vi "RS485通信实验.vi"   [LabVIEW 2011]
uses:
  <vilib>/STM32_DriverVI_Interface_F4/UART/UART Resource Name_F4.ctl
  <vilib>/STM32_DriverVI_Interface_F4/GPIO/PortX_in_F4.ctl
  <vilib>/STM32_DriverVI_Interface_F4/GPIO/pin_in_F4.ctl
  <vilib>/STM32_DriverVI_Interface_F4/GPIO/GPO_Mode_Interface_F4.ctl
  <vilib>/STM32_DriverVI_Interface_F4/LCD/Show_Mode_F4.ctl
  <vilib>/STM32_DriverVI_Interface_F4/LCD/Font_Size_F4.ctl
  <vilib>/STM32_DriverVI_Interface_F4/LCD/Brush Color_Index_F4.ctl
  <vilib>/eio/EIO_TerminalDirection.ctl
  <vilib>/STM32_DriverVI_Interface_F4/LCD/LCD_Init_F4.vi
  <vilib>/STM32_DriverVI_Interface_F4/GPIO_EIO/GPI_EIO_Inner_F4.vi
  <vilib>/eio/EIONode/EIONode.xnode
types:
  T1 = typedef "GPO_Mode_Interface_F4.ctl" = enum8{"Push-pull Output", "Open-drain Output"}
  T2 = typedef "pin_in_F4.ctl" = enum8{"P0", "P1", "P2", "P3", "P4", "P5", "P6", "P7", "P8", "P9", "P10", "P11", "P12", "P13", "P14", "P15"}
  T3 = typedef "PortX_in_F4.ctl" = enum8{"Port_A", "Port_B", "Port_C", "Port_D", "Port_E", "Port_F", "Port_G", "Port_H", "Port_I"}
  T4 = enum16{"1.0 bit", "0.5 bit", "2.0 bit", "1.5 bit"}
  T5 = enum16{"None parity", "Odd parity", "Even parity"}
  T6 = typedef "UART Resource Name_F4.ctl" = enum8{"COM 1", "COM 2", "COM 3", "COM 4", "COM 5", "COM 6"}
  T7 = typedef "STM32时钟倍频_F4.ctl" = u8
  T8 = typedef "Show_Mode_F4.ctl" = enum8{"非叠加显示", "叠加显示"}
  T9 = typedef "Font_Size_F4.ctl" = enum8{"Small_Font（12）", "Big_Font（16）"}
  T10 = typedef "Brush Color_Index_F4.ctl" = enum8{"White", "Black", "Blue", "Green_Blue", "Red", "Magenta（品红）", "Green", "Cyan（青色）", "Yellow", "Brown", "Brown_Red", "Gray", "Dark_Blue", "Light_Blue", "Gray_Blue", "Light_Green", "Light_Gray", "Light_Gray_Blue", "Light_Brown_Blue"}
  T11 = enum8{"P0", "P1", "P2", "P3", "P4", "P5", "P6", "P7", "P8", "P9", "P10", "P11", "P12", "P13", "P14", "P15"}
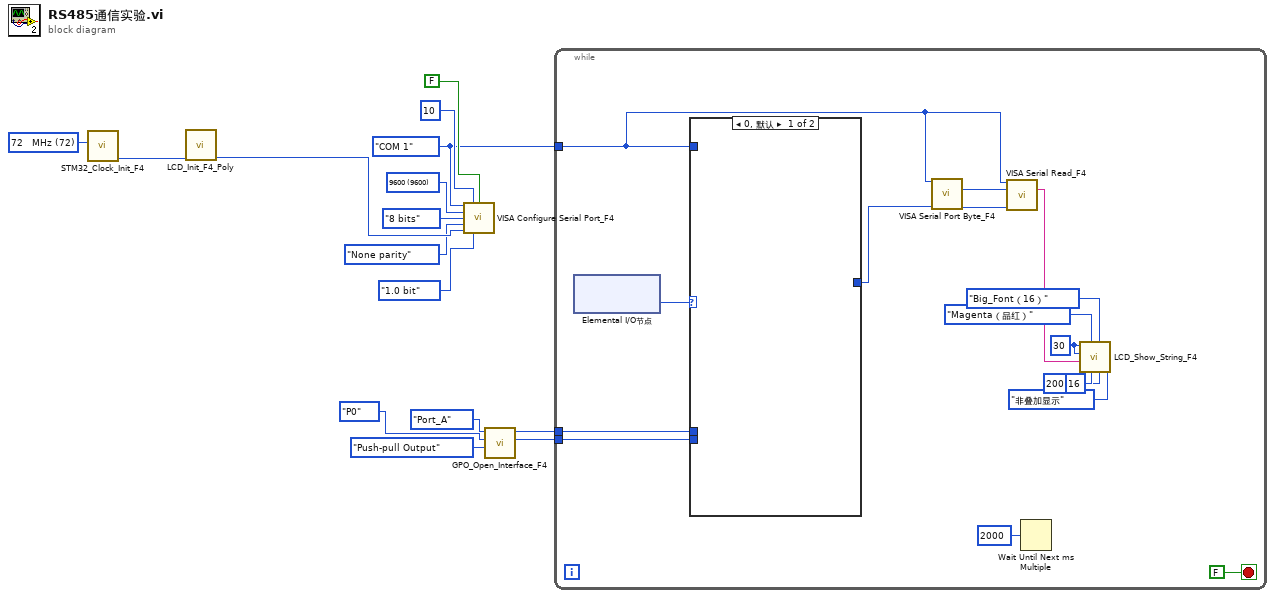
[diagram p0: block diagram]
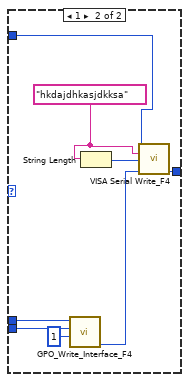
[diagram p2: hidden frame]
diagram:
  w12 = u32 9600 items=["4800"=4800, "9600"=9600, "14400"=14400, "19200"=19200, "38400"=38400, "115200"=115200] ("baud rate (9600)")
  w1 = UART_Resource_Name_F4."COM 1" ("VISA resource name")
  w15 = T7 72 items=["32   MHz"=32, "72   MHz"=72, "120 MHz"=120, "168 MHz"=168, "216 MHz"=216] ("STM32F4时钟倍频")
  n1 = call <vilib>:"STM32_Clock_Init_F4.vi"("STM32F4时钟倍频"=w15) -> ("err_out"=w14:u8)  [unwired: 10 in]
  n2 = call-poly <vilib>:"LCD_Init_F4_Poly.vi"("err_in"=w14) -> ("err_out"=w13:u8)  [unwired: 9 in, 1 out]
  n3 = call <vilib>:"VISA Configure Serial Port_F4.vi"("VISA resource name"=w1, "termination char\n(0xA = '\\n' = LF)"=u8 10 ("termination char\n(0xA = '\\n' = LF)"), "Enable Termination Char (T)"=FALSE, "baud rate (9600)"=w12, "data bits (8)"=enum16{"8 bits", "9 bits"}."8 bits", "parity (0:none)"=T5."None parity", "err in"=w13, "stop bits (10: 1 bit)"=T4."1.0 bit") -> ()  [unwired: 7 in, 1 out]
  n4 = call <vilib>:"GPO_Open_Interface_F4.vi"("mode"=GPO_Mode_Interface_F4."Push-pull Output", "pin_in"=pin_in_F4."P0", "PortX_in"=PortX_in_F4."Port_A") -> ("pin_out"=w2:u16, "PortX_out"=w3:u16)  [unwired: 6 in, 1 out]
  n5 = while {
    tunnel: w3 -> [w30]
    tunnel: w2 -> [w29]
    tunnel: w1 -> [w25]
    stop <- FALSE stop-if-true
    w19 = u16 30 ("X_Position")
    n6 = xnode "Elemental I/O节点"() -> ("KEY_UP"=w31:u8)  [unwired: 1 in, 1 out]
    n7 = case shown="0, 默认" w31 {
      tunnel: w25 -> [_ w37]
      tunnel: [_ w35] -> w28
      tunnel: w30 -> [_ w34]
      tunnel: w29 -> [_ w33]
      frame 0, Default {
      }
      frame 1 {
        w38 = "hkdajdhkasjdkksa"
        n8 = call <vilib>:"GPO_Write_Interface_F4.vi"("Level_Value"=u8 1, "pin_in"=w33, "PortX_in"=w34) -> ("err out"=w36:u8)  [unwired: 6 in, 2 out]
        n9 = String Length(string=w38) -> (length=w39:i32)
        n10 = call <vilib>:"VISA Serial Write_F4.vi"("VISA resource name"=w37, "字符串"=w38, "写入字节数"=w39, "err in"=w36) -> ("err out"=w35:u8)  [unwired: 11 in]
      }
    }
    n11 = call <vilib>:"VISA Serial Port Byte_F4.vi"("VISA resource name"=w25, "err in"=w28) -> ("串口字节数"=w26:u16, "err out"=w27:u8)  [unwired: 12 in]
    n12 = call <vilib>:"VISA Serial Read_F4.vi"("VISA resource name"=w25, "读取字节数"=w26, "err in"=w27) -> ("字符串"=w20:string)  [unwired: 10 in, 2 out]
    n13 = Wait Until Next ms Multiple(millisecond multiple=u32 2000 ("毫秒倍数")) -> ()  [unwired: 1 out]
    n14 = call <vilib>:"LCD_Show_String_F4.vi"("Show_Mode"=Show_Mode_F4."非叠加显示", "Height"=u16 16, "Font_Size"=Font_Size_F4."Big_Font（16）", "Width"=u16 200, "Brush Color"=Brush_Color_Index_F4."Magenta（品红）", "String"=w20, "Y_Position"=w19, "X_Position"=w19) -> ()  [unwired: 3 in, 1 out]
  }
